vi "CliSetConnectionType.vi"(0 "ref in":u64, 7 "ConnectionType":u16(ring)=1 items=["PG"=1, "OP"=2, "S7 Basic"=3], 11 "error in (no error)":errorcluster) -> (4 "ref out":u64, 6 "Result":i32, 15 "error out":errorcluster)   [LabVIEW 2014, in "Snap7.lvlib"]
uses:
  Snap7.lvlib
  windows/lv_snap7.dll
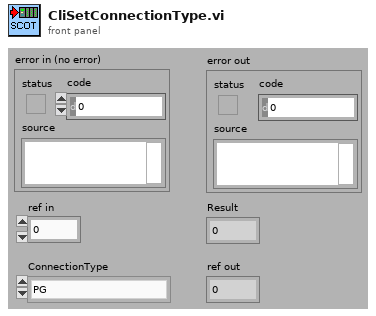
[diagram p1: front panel]
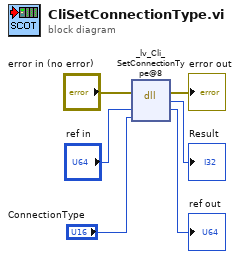
[diagram p0: block diagram]
diagram:
  n1 = dll-call lib="D:/Libraries/Snap7_1.4.2/LabVIEW/lib/windows/lv_snap7.dll" fn="_lv_Cli_SetConnectionType@8"(error in="error in (no error)", "Client"="ref in", "ConnectionType"="ConnectionType") -> (error out=→"error out":errorcluster, "return type"=→"Result":i32, "Client"=→"ref out":u64)  [unwired: 3 in, 1 out]
